vi "Set_DeferUpdates.vi"(7 "Front Panel":refnum<vi>, 8 "error in (no error)":errorcluster, 9 "Defer Panel Updates":bool, 10 "Control Label":string, 11 "CtlLookup In":T1) -> (0 "error out":errorcluster, 2 "Front Panel Out":refnum<vi>, 3 "CtlLookup Out":T1)   [LabVIEW 2020, in "CtlReferences.lvlib" / "CtlReferences.lvclass"]
uses:
  CtlReferences.lvclass
  CtlReferences.lvclass/CtlReferences.ctl
  TypeDefs/CtlLookup.ctl
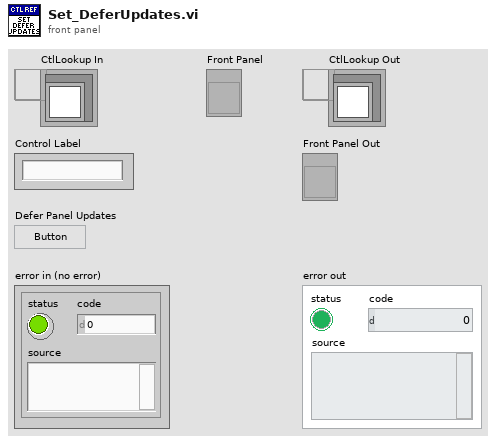
[diagram p1: front panel]
types:
  T1 = typedef "CtlReferences.lvlib/CtlReferences.lvclass/CtlLookup.ctl" = refnum<data-value>
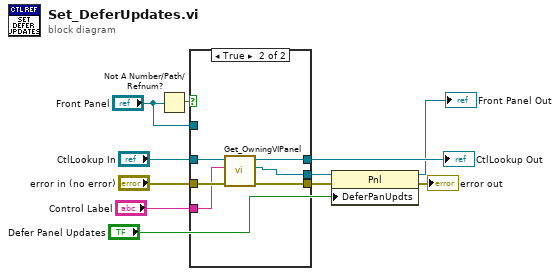
[diagram p0: block diagram]
diagram:
  n1 = Not A Number/Path/Refnum?(number/path/refnum="Front Panel") -> (NaN/Path/Refnum?=w3:bool)
  n2 = case shown="True" w3 {
    tunnel: "CtlLookup In" -> [w13 w20]
    tunnel: "error in (no error)" -> [w12 w19]
    tunnel: [w13 w18] -> w9
    tunnel: [w12 w17] -> w8
    tunnel: [w14 w16] -> w5
    tunnel: "Control Label" -> [_ w15]
    tunnel: "Front Panel" -> [w14 _]
    frame False {
    }
    frame True {
      n3 = call "Get_OwningVIPanel.vi"("error in (no error)"=w19, "Control Label"=w15, "CtlLookup In"=w20) -> ("error out"=w17:errorcluster, "Front Panel"=w16:refnum<vi>, "CtlLookup Out"=w18:T1)  [unwired: 5 in, 1 out]
    }
  }
  "CtlLookup Out" <- w9
  n4 = property class="Pnl"(reference=w5, error in=w8, "DeferPanUpdts"="Defer Panel Updates") -> (reference out=→"Front Panel Out":refnum<vi>, error out=→"error out":errorcluster)
